vi "GUI_Cascade.vi"() -> ()   [LabVIEW 2013]
uses:
  Shared/GUI_Template/GUI_master/tcp_new_data_event.ctl
  Shared/GUI_Template/GUI_master/tcp new data cluster.ctl
  <vilib>/vision/NI_Vision_Development_Module.lvlib
panel:
  out "Histogram Report":T1 {"Standard  Variation" format="%.2f"; "Mean Value" format="%.2f"; "Interval Width" format="%.2f"; "Starting Value" format="%.2f"; "Maximal Value" format="%.2f"; "Minimal Value" format="%.2f"}
  in  "Number of histogram bins":i32=256
  out "Mean Value":sgl format="%.2f"
  in  "localsavingpath::1":path caption="LocalSavingPath"
  in  "STOP":bool
  out "Lineout":dbl[](graph)
  in  "exposure::1":dbl=40.0 caption="Exposure" min=0.0 max=20000.0
  in  "ADCGain::1":dbl=1.0 caption="ADC Gain" min=0.0 max=2000.0
  in  "AvalancheGain::1":dbl=3000.0 caption="Avalanche Gain" min=0.0 max=10000.0
  in  "Refresh Button":bool
  in  "save::1":bool caption="Save"
  in  "FastADC::1":bool caption="FastADC"
  in  "ROI.Xend::1":dbl=512.0 caption="ROI.Xend" min=1.0 max=512.0
  in  "ROI.Yend::1":dbl=512.0 caption="ROI.Yend" min=1.0 max=512.0
  in  "ROI.Ystart::1":dbl=1.0 caption="ROI.Ystart" min=1.0 max=512.0
  in  "ROI.Xstart::1":dbl=1.0 caption="ROI.Xstart" min=1.0 max=512.0
  in  "ROI.Ybinning::1":dbl=1.0 caption="Y binning" min=1.0 max=512.0
  in  "ROI.Xbinning::1":dbl=1.0 caption="X binning" min=1.0 max=512.0
  in  "trigger::1":T2(ring)=enum."Trigger First (PM only)" caption="Trigger"
  out "image::1":T3(plugin-control) caption="Casca512"
  out "Histogram":T4(graph)
  in  "GUIdevice 1":string="Cascade512"
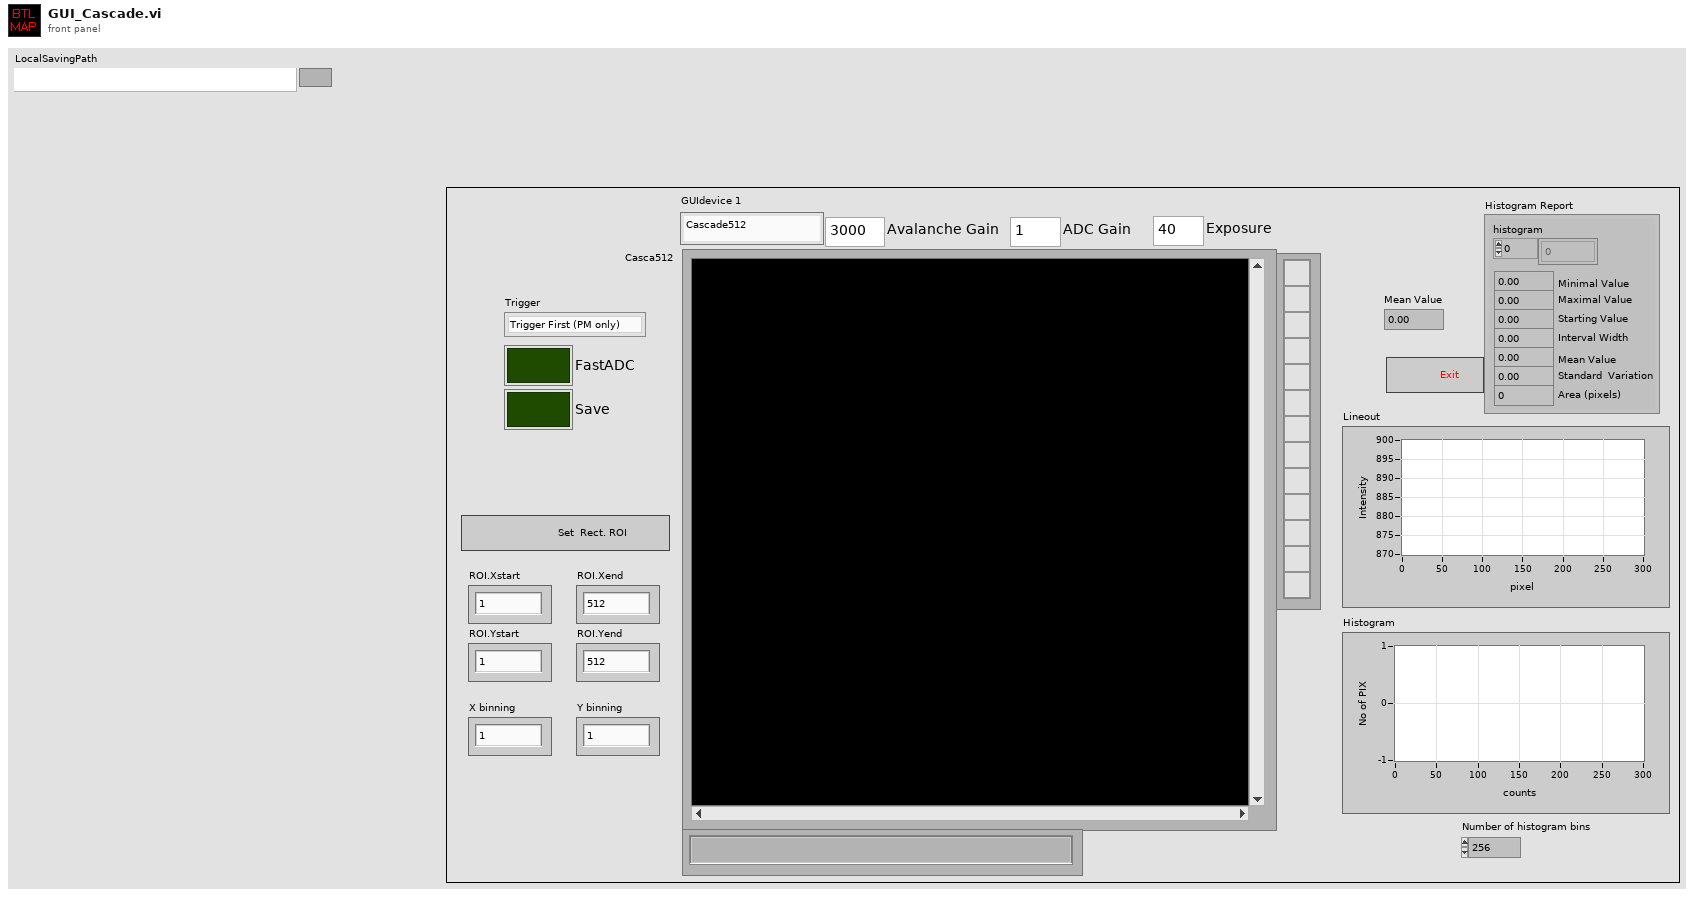
[diagram p1: front panel]
types:
  T1 = cluster{"histogram":u32[], "Minimal Value":sgl, "Maximal Value":sgl, "Starting Value":sgl, "Interval Width":sgl, "Mean Value":sgl, "Standard  Variation":sgl, "Area (pixels)":i32}
  T2 = enum32{"N/A", "Free Run/Timed", "Trigger First (PM only)", "Ext Sync/Strobed", "Bulb (PM only)", "Variable Exp (PM only)", "Flash Mode (PM only)"}
  T3 = typedef "IMAQ Image.ctl" = refnum<image>
  T4 = cluster{"Starting Value":sgl, "Incremental Value":sgl, "Histogram":u32[]}
  T5 = enum32{"invalid app kind", "Development System", "Run Time System", "Student Edition", "Embedded LabVIEW", "Evaluation", "Custom"}
  T6 = typedef "tcp_new_data_event.ctl" = refnum<user-event>
  T7 = typedef "tcp new data cluster.ctl" = cluster{"EventEnum":enum16{"new data", "connection status update"}, "Device name":string}
  T8 = enum32{"Invalid", "Standard", "Closed", "Hidden", "Minimized", "Maximized"}
  T9 = cluster{"Global Rectangle":i32[], "Contours":cluster{"Contour Type":u32, "ROI Type":u32, "Points":i32[]}[]}
  T10 = typedef "IMAQ Line" = cluster{"Start X":i32, "Start Y":i32, "End X":i32, "End Y":i32}
  T11 = typedef "IMAQ Rectangle" = cluster{"Left":i32, "Top":i32, "Right":i32, "Bottom":i32, "Rotation":dbl}
  T12 = cluster{"Core":cluster{"Current VI Reference":refnum<vi>, "Close Panel on Exit?":bool}, "Your Boolean data":bool, "Your string data":string, "SuperGUI":cluster{"STOP queue":refnum<queue>, "SuperGUI ref":refnum<vi>}, "New Image":T3, "tcp data event":T6}
  T13 = typedef "Image Type" = u32
  T14 = cluster{"STOP queue":refnum<queue>, "SuperGUI ref":refnum<vi>}
  T15 = cluster{"Current VI Reference":refnum<vi>, "Close Panel on Exit?":bool}
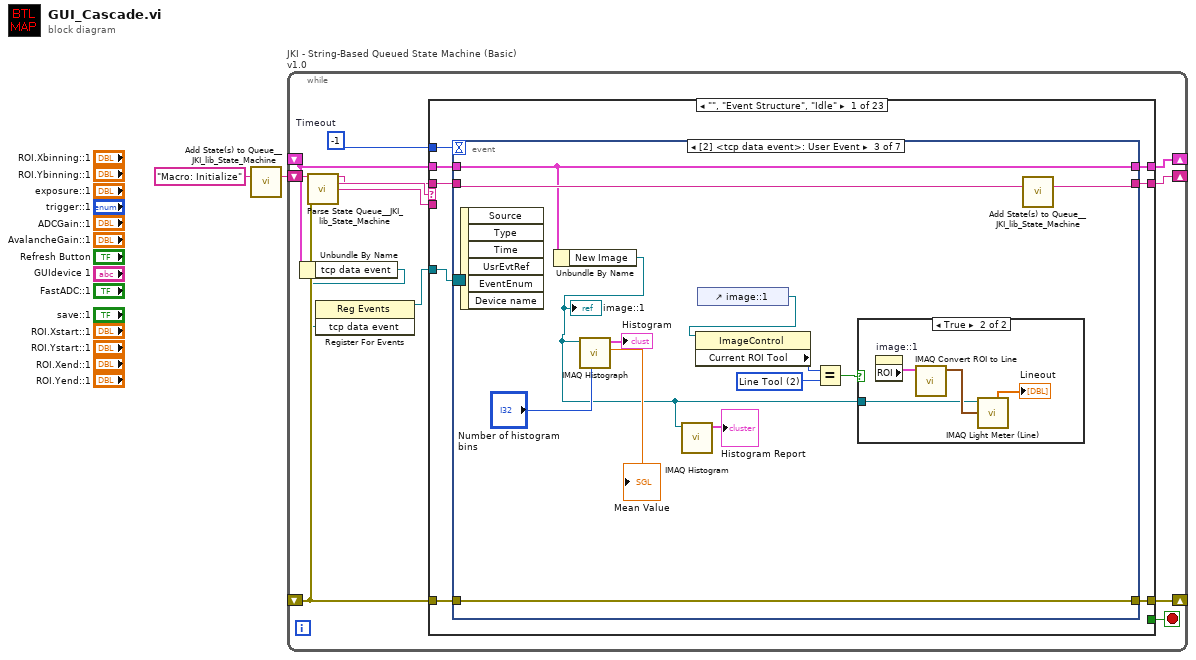
[diagram p0: block diagram]
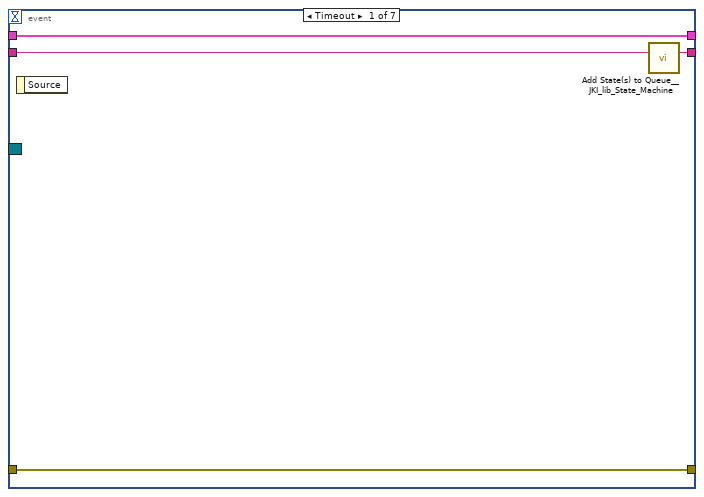
[diagram p2: hidden frame]
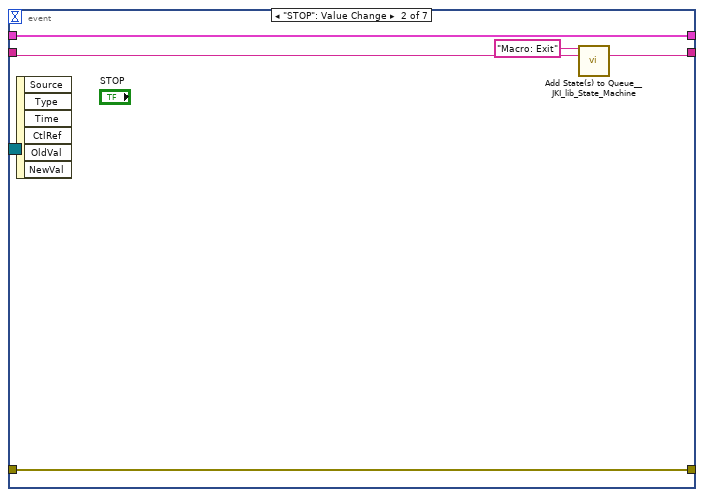
[diagram p3: hidden frame]
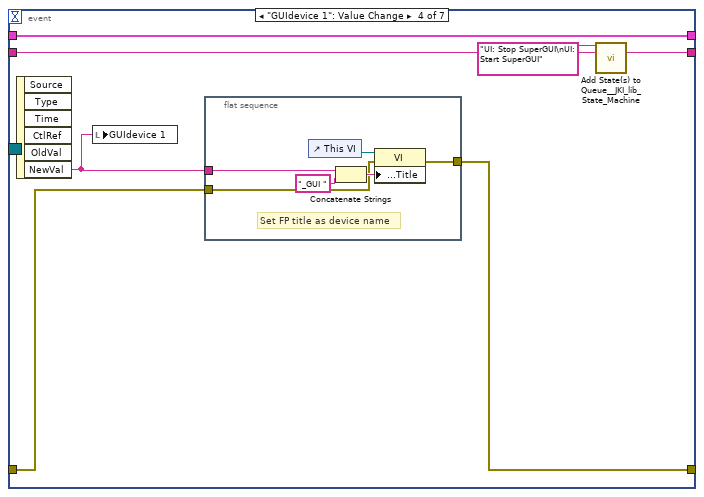
[diagram p5: hidden frame]
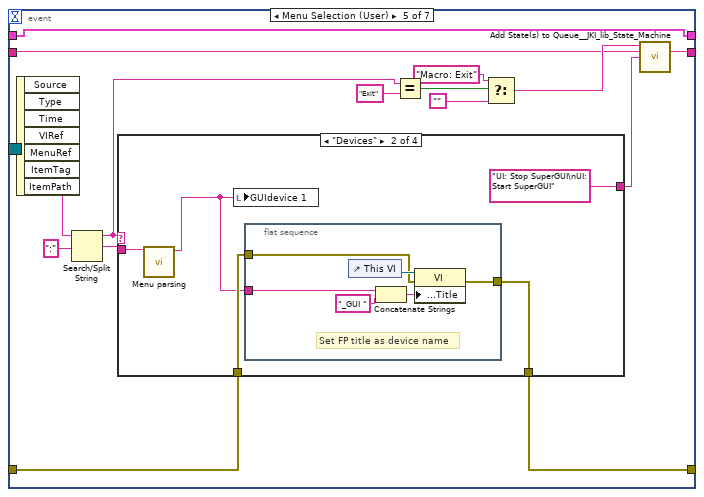
[diagram p6: hidden frame]
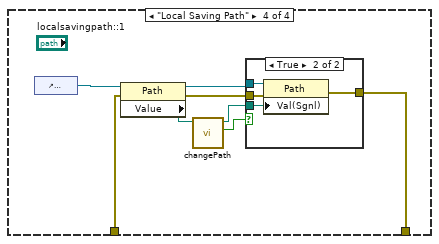
[diagram p9: hidden frame]
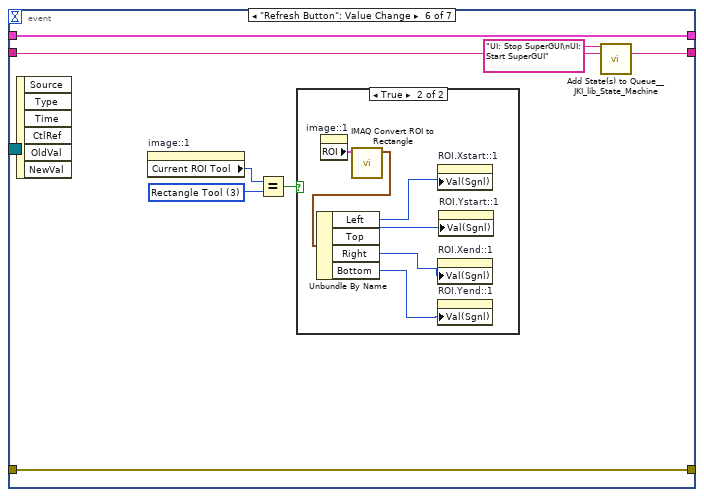
[diagram p11: hidden frame]
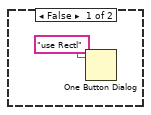
[diagram p12: hidden frame]
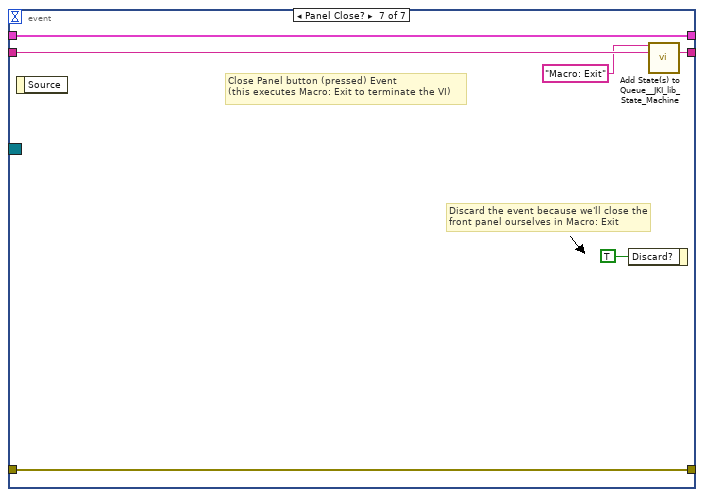
[diagram p13: hidden frame]
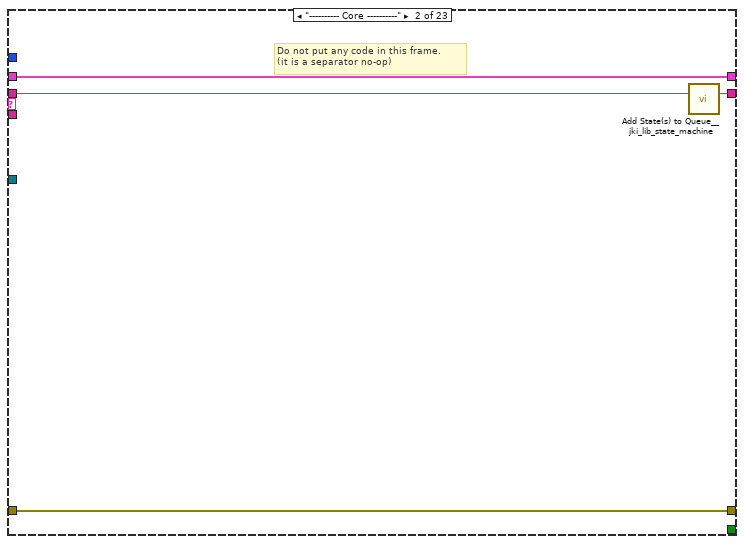
[diagram p14: hidden frame]
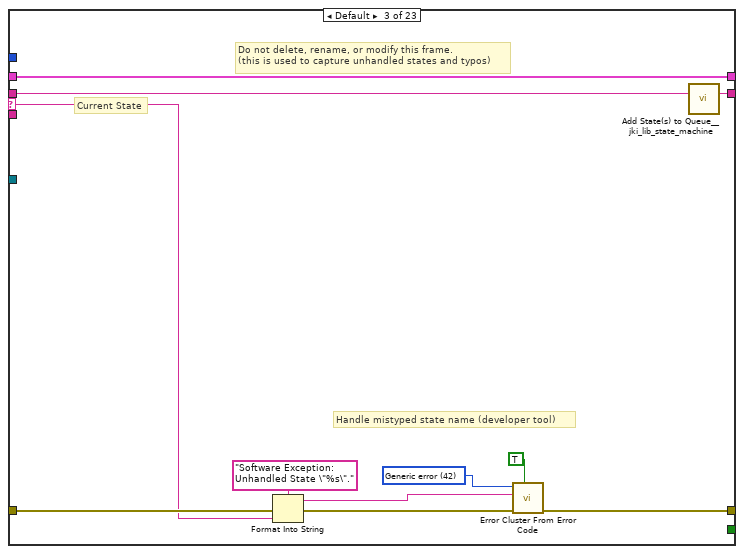
[diagram p15: hidden frame]
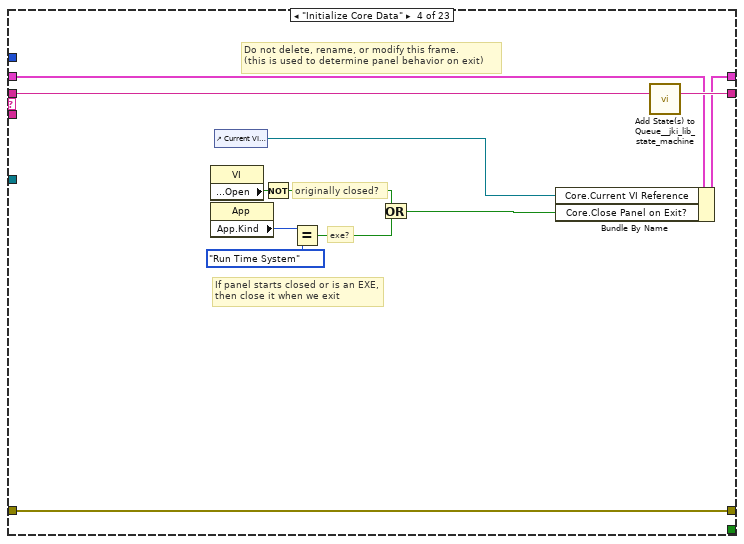
[diagram p16: hidden frame]
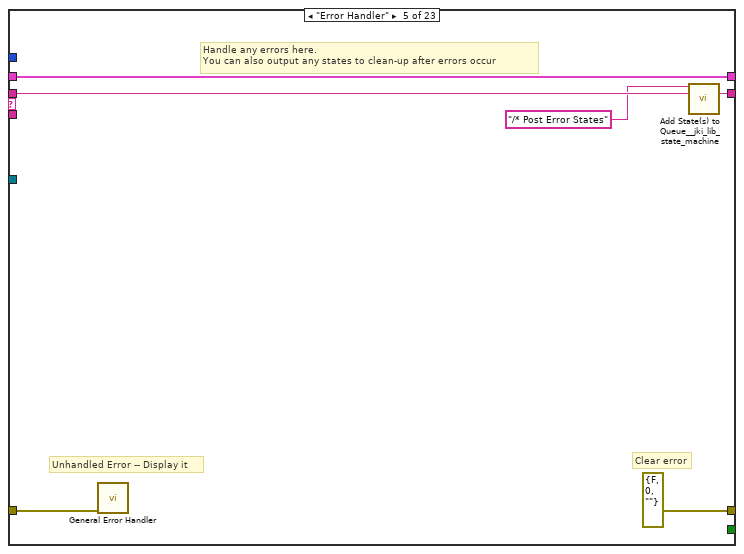
[diagram p17: hidden frame]
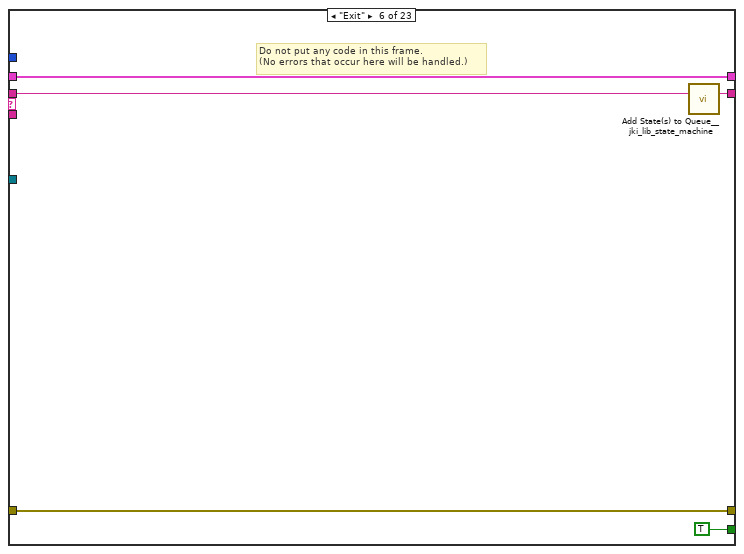
[diagram p18: hidden frame]
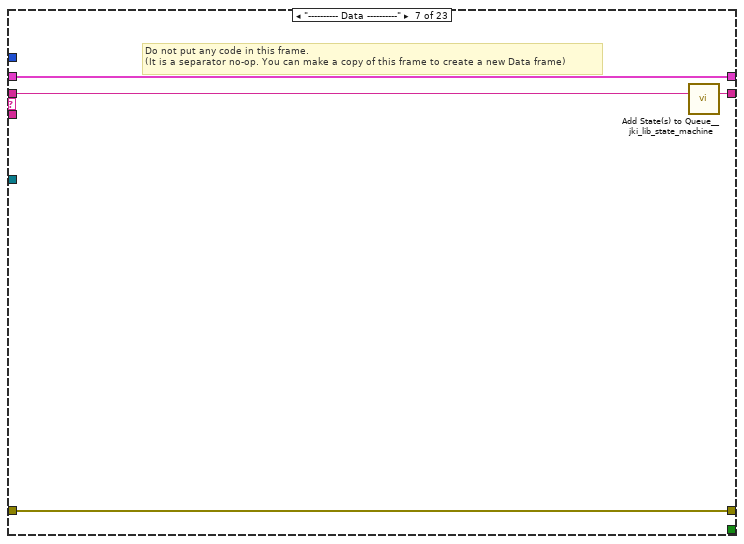
[diagram p19: hidden frame]
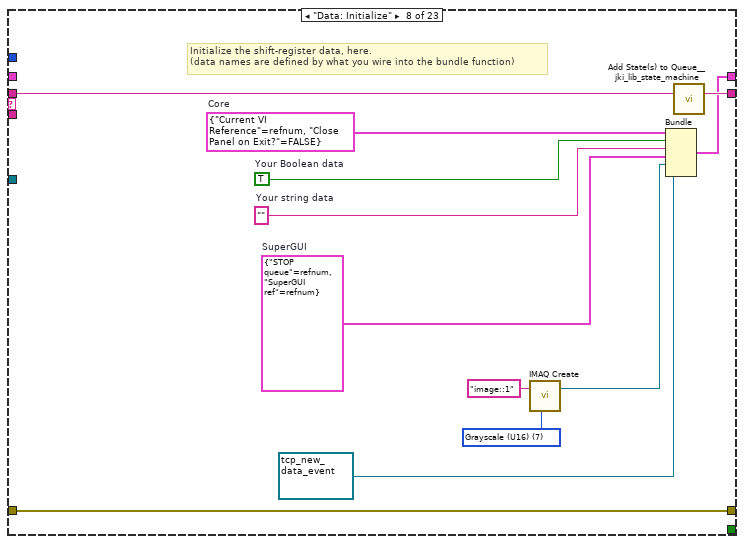
[diagram p20: hidden frame]
diagram:
  n1 = call <vilib>:"Add State(s) to Queue__JKI_lib_State_Machine.vi"("State(s) in (\"\")"="Macro: Initialize") -> ("States Out"=w2:string)  [unwired: 14 in]
  n2 = while "JKI - String-Based Queued State Machine (Basic) v1.0" {
    shift-right: [w8] -> _
    shift-left: _ -> [w5]
    shift-right: [w11] -> _
    shift-left: _ -> [w6]
    shift-right: [w10] -> _
    shift-left: w2 -> [w12]
    stop <- w9 stop-if-true
    w7 = -1  # Timeout
    n3 = Unbundle By Name(w5) -> ("tcp data event"=w4:T6)
    n4 = call <vilib>:"Parse State Queue__JKI_lib_State_Machine.vi"("State Queue"=w12, "Error In (no error)"=w6) -> ("Remaining States"=w14:string, "Current State"=w15:string, "Arguments"=w13:string)  [unwired: 11 in]
    n5 = register-events(w4) -> (reference out=w3:refnum<event-registration>)  [unwired: 2 in, 1 out]
    n6 = case shown="\"\", \"Event Structure\", \"Idle\"" w15 {
      selector: w15 -> [_ _ w129 _ _ _ _ _ _ _ _ _ _ _ _ _ _ _ _ _ _ _ _]
      tunnel: w14 -> [w23 w128 w133 w151 w157 w162 w166 w178 w184 w188 w193 w198 w236 w270 w278 w284 w295 w321 w326 w336 w340 w344 w348]
      tunnel: w13 -> [_ _ _ _ _ _ _ _ _ _ _ _ _ _ _ w279 w289 _ _ _ _ _ _]
      tunnel: w5 -> [w21 w125 w131 w142 w154 w160 w163 _ w179 w185 w191 w196 w234 w261 w273 w282 w291 w318 w323 w333 w337 w341 w345]
      tunnel: [w20 w126 w135 w148 errorcluster {"status"=FALSE, "code"=0, "source"=""} ("error out") w159 w164 w175 w180 w186 w189 w194 w231 w255 w271 w280 w292 w319 w324 w334 w338 w342 w346] -> w11
      tunnel: w6 -> [w19 w126 w134 w148 w153 w159 w164 w175 w181 w186 w190 w195 w232 w256 w272 w281 w293 w319 w324 w334 w338 w342 w346]
      tunnel: [w22 w127 w132 w150 w156 w161 w165 w177 w183 w187 w192 w197 w235 w269 w277 w283 w294 w320 w325 w335 w339 w343 w347] -> w10
      tunnel: [_ _ _ _ _ TRUE _ _ _ _ _ _ _ _ _ _ _ _ _ _ _ _ _] -> w9
      tunnel: [w18 w125 w131 w149 w154 w160 w163 w176 w179 w185 w191 w196 w234 w260 w273 w282 w291 w318 w323 w333 w337 w341 w345] -> w8
      tunnel: w7 -> [w17 _ _ _ _ _ _ _ _ _ _ _ _ _ _ _ _ _ _ _ _ _ _]
      tunnel: w3 -> [w16 _ _ _ _ _ _ _ _ _ _ _ _ _ _ _ _ _ _ _ _ _ _]
      frame "", "Event Structure", "Idle" {
        n7 = event shown="[2] <tcp data event>: User Event" {
          selector: w16 -> [_ _ _ _ _ _ _]
          dyn-events: _ -> [_ _ _ _ _ _ _]
          timeout: w17 -> [_ _ _ _ _ _ _]
          tunnel: w23 -> [w27 w30 w44 w53 w71 w109 w124]
          tunnel: [w26 w29 w43 w52 w70 w108 w123] -> w22
          tunnel: w21 -> [w24 w32 w38 w56 w77 w111 w121]
          tunnel: [w25 w31 w45 w54 w64 w110 w122] -> w20
          tunnel: w19 -> [w25 w31 w45 w55 w65 w110 w122]
          tunnel: [w24 w32 w38 w56 w77 w111 w121] -> w18
          event Timeout {
            n8 = event-data() -> ()  [unwired: 1 in, 1 out]
            n9 = call <vilib>:"Add State(s) to Queue__JKI_lib_State_Machine.vi"("State(s) in (\"\")"=w27) -> ("States Out"=w26:string)  [unwired: 14 in]
          }
          event "STOP": Value Change {
            n10 = event-data() -> ()  [unwired: 1 in, 6 out]
            n11 = call <vilib>:"Add State(s) to Queue__JKI_lib_State_Machine.vi"("State(s) in Front (\"\")"="Macro: Exit", "State(s) in (\"\")"=w30) -> ("States Out"=w29:string)  [unwired: 13 in]
          }
          event User Event {
            w41 = u32 2 items=["Zoom Tool"=8, "Selection Tool"=0, "Pan Tool"=9, "Point Tool"=1, "Line Tool"=2, "Rectangle Tool"=3, "Rotated Rectangle Tool"=12, "Polyline Tool"=10, "Polygon Tool"=5, "Freehand Tool"=11, "Closed Freehand Tool"=6, "Ellipse Tool"=4, "Annulus Tool"=7] ("Current ROI Tool")
            n12 = event-data() -> ()  [unwired: 1 in, 6 out]
            n13 = Unbundle By Name(w38) -> ("New Image"=w34:T3)
            "image::1" <- w34
            n14 = call "IMAQ Histograph"("Number of Classes"="Number of histogram bins", "Image"=w34) -> ("Mean Value"=→"Mean Value":sgl, "Histogram Graph"=→"Histogram":T4)  [unwired: 6 in, 2 out]
            n15 = call "IMAQ Histogram"("Image"=w34) -> ("Histogram Report"=→"Histogram Report":T1)  [unwired: 9 in, 1 out]
            n16 = control-ref of="image::1"() -> (w37:refnum<vi>)
            n17 = property on="Property Node" class="ImageControl"(reference=w37) -> ("Current ROI Tool"=w40:u32)  [unwired: 1 in, 2 out]
            n18 = Equal?(x=w40, y=w41) -> (x = y?=w42:bool)
            n19 = case shown="True" w42 {
              tunnel: w34 -> [_ w47]
              frame False {
              }
              frame True {
                n20 = property on="image::1" class="ImageControl"() -> ("ROI"=w49:T9)  [unwired: 2 in, 2 out]
                n21 = call "IMAQ Convert ROI to Line"("ROI Descriptor"=w49) -> ("Line"=w48:T10)  [unwired: 8 in, 1 out]
                n22 = call "IMAQ Light Meter (Line)"("Line"=w48, "Image"=w47) -> ("Line Profile"=→"Lineout":dbl[])  [unwired: 5 in, 4 out]
              }
            }
            n23 = call <vilib>:"Add State(s) to Queue__JKI_lib_State_Machine.vi"("State(s) in (\"\")"=w44) -> ("States Out"=w43:string)  [unwired: 14 in]
          }
          event "GUIdevice 1": Value Change {
            n24 = event-data() -> ("NewVal"=w50:string)  [unwired: 1 in, 5 out]
            n25 = local write "GUIdevice 1"(w50) -> ()
            n26 = flat-sequence {
              tunnel: [w59] -> w54
              tunnel: w55 -> [w58]
              tunnel: w50 -> [w57]
              frame #0 {
                # "Set FP title as device name"
                n27 = control-ref of="This VI"() -> (w62:refnum<vi>)
                n28 = Concatenate Strings(w57, "_GUI ") -> (w61:string)
                n29 = property class="VI"(reference=w62, error in=w58, "Front Panel.Title"=w61) -> (error out=w59:errorcluster)  [unwired: 1 out]
              }
            }
            n30 = call <vilib>:"Add State(s) to Queue__JKI_lib_State_Machine.vi"("State(s) in Front (\"\")"="UI: Stop SuperGUI\nUI: Start SuperGUI", "State(s) in (\"\")"=w53) -> ("States Out"=w52:string)  [unwired: 13 in]
          }
          event Menu Selection (User) {
            n31 = event-data() -> ("ItemPath"=w67:string)  [unwired: 1 in, 6 out]
            n32 = Search/Split String(string=w67, search string/char (-)=":") -> (substring before match=w63:string, match + rest of string=w66:string)  [unwired: 1 in, 1 out]
            n33 = case shown="\"Devices\"" w63 {
              tunnel: w66 -> [_ w83 _ _]
              tunnel: w65 -> [w78 w82 w90 w93]
              tunnel: [w78 w81 w90 w92] -> w64
              tunnel: [_ "UI: Stop SuperGUI\nUI: Start SuperGUI" _ _] -> w69
              frame "", Default {
              }
              frame "Devices" {
                n34 = call "Menu parsing.vi"("ItemPath"=w83) -> ("ItemPath"=w79:string)  [unwired: 9 in, 1 out]
                n35 = local write "GUIdevice 1"(w79) -> ()
                n36 = flat-sequence {
                  tunnel: [w86] -> w81
                  tunnel: w82 -> [w85]
                  tunnel: w79 -> [w84]
                  frame #0 {
                    # "Set FP title as device name"
                    n37 = control-ref of="This VI"() -> (w89:refnum<vi>)
                    n38 = Concatenate Strings(w84, "_GUI ") -> (w88:string)
                    n39 = property class="VI"(reference=w89, error in=w85, "Front Panel.Title"=w88) -> (error out=w86:errorcluster)  [unwired: 1 out]
                  }
                }
              }
              frame "Exit" {
              }
              frame "Local Saving Path" {
                n40 = control-ref of="localsavingpath::1"() -> (w94:refnum<vi>)
                n41 = property class="Path"(reference=w94, error in=w93) -> (reference out=w96:refnum<vi>, error out=w91:errorcluster, "Value"=w95:path)
                n42 = call "changePath.vi"("Local Saving in (h)"=w95) -> ("change (h)"=w97:bool, "Local Saving out (h)"=w98:path)  [unwired: 9 in]
                n43 = case shown="True" w97 {
                  tunnel: w96 -> [_ w103]
                  tunnel: w98 -> [_ w102]
                  tunnel: [w99 w101] -> w92
                  tunnel: w91 -> [w99 w100]
                  frame False {
                  }
                  frame True {
                    n44 = property class="Path"(reference=w103, error in=w100, "Val(Sgnl)"=w102) -> (error out=w101:errorcluster)  [unwired: 1 out]
                  }
                }
              }
            }
            n45 = Equal?(x=w63, y="Exit") -> (x = y?=w75:bool)
            n46 = Select(t="Macro: Exit", s=w75, f="") -> (s? t:f=w72:string)
            n47 = call <vilib>:"Add State(s) to Queue__JKI_lib_State_Machine.vi"("State(s) in Front (\"\")"=w72, "State(s) in (\"\")"=w71, "State(s) at Back (\"\")"=w69) -> ("States Out"=w70:string)  [unwired: 12 in]
          }
          event "Refresh Button": Value Change {
            w105 = u32 3 items=["Zoom Tool"=8, "Selection Tool"=0, "Pan Tool"=9, "Point Tool"=1, "Line Tool"=2, "Rectangle Tool"=3, "Rotated Rectangle Tool"=12, "Polyline Tool"=10, "Polygon Tool"=5, "Freehand Tool"=11, "Closed Freehand Tool"=6, "Ellipse Tool"=4, "Annulus Tool"=7] ("Current ROI Tool")
            n48 = event-data() -> ()  [unwired: 1 in, 6 out]
            n49 = property on="image::1" class="ImageControl"() -> ("Current ROI Tool"=w106:u32)  [unwired: 2 in, 2 out]
            n50 = Equal?(x=w106, y=w105) -> (x = y?=w104:bool)
            n51 = case shown="True" w104 {
              frame False {
                n52 = One Button Dialog(message="use Rectl") -> ()  [unwired: 1 in, 1 out]
              }
              frame True {
                n53 = property on="image::1" class="ImageControl"() -> ("ROI"=w118:T9)  [unwired: 2 in, 2 out]
                n54 = call "IMAQ Convert ROI to Rectangle"("ROI Descriptor"=w118) -> ("Rectangle"=w117:T11)  [unwired: 8 in, 1 out]
                n55 = Unbundle By Name(w117) -> ("Left"=w116:i32, "Top"=w115:i32, "Right"=w114:i32, "Bottom"=w113:i32)
                n56 = property on="ROI.Xstart::1" class="DigNum (strict)"("Val(Sgnl)"=w116) -> ()  [unwired: 2 in, 2 out]
                n57 = property on="ROI.Xend::1" class="DigNum (strict)"("Val(Sgnl)"=w114) -> ()  [unwired: 2 in, 2 out]
                n58 = property on="ROI.Yend::1" class="DigNum (strict)"("Val(Sgnl)"=w113) -> ()  [unwired: 2 in, 2 out]
                n59 = property on="ROI.Ystart::1" class="DigNum (strict)"("Val(Sgnl)"=w115) -> ()  [unwired: 2 in, 2 out]
              }
            }
            n60 = call <vilib>:"Add State(s) to Queue__JKI_lib_State_Machine.vi"("State(s) in Front (\"\")"="UI: Stop SuperGUI\nUI: Start SuperGUI", "State(s) in (\"\")"=w109) -> ("States Out"=w108:string)  [unwired: 13 in]
          }
          event Panel Close? {
            # "Discard the event because we'll close the front panel ourselves in Macro: Exit"
            # "Close Panel button (pressed) Event\n(this executes Macro: Exit to terminate the VI)"
            n61 = event-data() -> ()  [unwired: 1 in, 1 out]
            n62 = event-data("Discard?"=TRUE) -> ()  [unwired: 1 in, 1 out]
            n63 = call <vilib>:"Add State(s) to Queue__JKI_lib_State_Machine.vi"("State(s) in Front (\"\")"="Macro: Exit", "State(s) in (\"\")"=w124) -> ("States Out"=w123:string)  [unwired: 13 in]
          }
        }
      }
      frame "---------- Core ----------" {
        # "Do not put any code in this frame.\n(it is a separator no-op)"
        n64 = call <vilib>:"Add State(s) to Queue__jki_lib_state_machine.vi"("State(s) in (\"\")"=w128) -> ("States Out"=w127:string)  [unwired: 14 in]
      }
      frame Default {
        w138 = 42 items=["No error", "Argument error", "Memory is full", "Out of zone", "End of file", "File already open", "Generic file I/O error", "File not found", "File permission error", "Disk is full", "Duplicate path", "Too many files open", "System feature not enabled", "Resource file not found", "Cannot add resource", "Resource not found", "Image not found", "Image memory error", "Pen does not exist", "Config type invalid", "Config token not found", "Config parse error", "Config memory error", "Bad external code format", "Bad external code offset", "External code not present", "Null window", "Destroy window error", "Null menu", "Print aborted", "Bad print record", "Print driver error", "Windows error during printing", "Memory error during printing", "Print dialog error", "Generic print error", "Invalid device refnum", "Device not found", "Device parameter error", "Device unit error", "Cannot open device", "Device call aborted", "Generic error", "Cancelled by user", "Object ID too low", "Object ID too high", "Object not in heap", "Unknown heap", "Unknown object (invalid DefProc)", "Unknown object (DefProc not in table)", "Message out of range", "Invalid (null) method", "Unknown message", "Manager call not supported", "Bad address", "Network operation in progress", "Network operation timed out", "Connection is busy", "Network attribute not supported", "Network error", "Address in use", "System out of memory", "Connection aborted", "Connection refused", "Not connected", "Already connected", "Connection closed", "Initialization error (interapplication manager)", "Bad occurrence", "Wait on unbound occurrence handler", "Occurrence queue overflow", "Datalog type conflict", "Unused", "Unrecognized type (interapplication manager)", "Memory corrupt", "Failed to make temporary DLL", "Old CIN version", "Drag socket not found", "Failed to load drop-object", "Failed to register OLE object", "Failed to release OLE object", "Format specifier type mismatch", "Unknown format specifier", "Too few format specifiers", "Too many format specifiers", "Scan failed", "Newer CIN version", "Error converting to variant", "Runtime menu error", "Password tampered", "Variant attribute not found", "Incompatible variant data type", "Event data is not available", "Event Store is not present", "Occurrence is not found", "Event Queue is not created", "Event info is not available", "Refnum passed is NULL", "Error retrieving Class GUID", "Error retrieving CoClass GUID", "Error retrieving TypeLib GUID.", "Bad built application magic bytes.", "Specific driver is different from the specific driver associated with the Logical Name.", "There is no session opened to the class driver.", "Max Error", "MAX - Error with config objects", "MAX - Error loading configuration", "MAX - Group not supported"]
        # "Current State"
        # "Do not delete, rename, or modify this frame.\n(this is used to capture unhandled states and typos)"
        # "Handle mistyped state name (developer tool)"
        n65 = Format Into String(format string="Software Exception: Unhandled State \"%s\"." ("message"), error in=w134, w129) -> (resulting string=w137:string, error out=w136:errorcluster)  [unwired: 1 in]
        n66 = call <vilib>:"Error Cluster From Error Code.vi"("show call chain? (False)"=TRUE, "error in (no error)"=w136, "error message (\"\")"=w137, "error code (0)"=w138) -> ("error out"=w135:errorcluster)  [unwired: 5 in]
        n67 = call <vilib>:"Add State(s) to Queue__jki_lib_state_machine.vi"("State(s) in (\"\")"=w133) -> ("States Out"=w132:string)  [unwired: 14 in]
      }
      frame "Initialize Core Data" {
        # "Do not delete, rename, or modify this frame.\n(this is used to determine panel behavior on exit)"
        # "originally closed?"
        # "exe?"
        # "If panel starts closed or is an EXE, then close it when we exit"
        n68 = property class="VI"() -> ("Front Panel.Open"=w147:bool)  [unwired: 2 in, 2 out]
        n69 = property class="App"() -> ("App.Kind"=w146:T5)  [unwired: 2 in, 2 out]
        n70 = control-ref of="Current VI Reference"() -> (w140:refnum<vi>)
        n71 = Not(x=w147) -> (.not. x?=w144:bool)
        n72 = Equal?(x=w146, y=T5."Run Time System" ("Application:Kind")) -> (x = y?=w143:bool)
        n73 = Or(x=w144, y=w143) -> (x .or. y?=w141:bool)
        n74 = Bundle By Name(cluster=w142, "Core.Current VI Reference"=w140, "Core.Close Panel on Exit?"=w141) -> (w149:T12)
        n75 = call <vilib>:"Add State(s) to Queue__jki_lib_state_machine.vi"("State(s) in (\"\")"=w151) -> ("States Out"=w150:string)  [unwired: 14 in]
      }
      frame "Error Handler" {
        # "Unhandled Error -- Display it"
        # "Handle any errors here.\nYou can also output any states to clean-up after errors occur"
        # "Clear error"
        n76 = call <vilib>:"General Error Handler.vi"("error in (no error)"=w153) -> ()  [unwired: 10 in, 5 out]
        n77 = call <vilib>:"Add State(s) to Queue__jki_lib_state_machine.vi"("State(s) in Front (\"\")"="/* Post Error States", "State(s) in (\"\")"=w157) -> ("States Out"=w156:string)  [unwired: 13 in]
      }
      frame "Exit" {
        # "Do not put any code in this frame.\n(No errors that occur here will be handled.)"
        n78 = call <vilib>:"Add State(s) to Queue__jki_lib_state_machine.vi"("State(s) in (\"\")"=w162) -> ("States Out"=w161:string)  [unwired: 14 in]
      }
      frame "---------- Data ----------" {
        # "Do not put any code in this frame.\n(It is a separator no-op. You can make a copy of this frame to create a new Data frame)"
        n79 = call <vilib>:"Add State(s) to Queue__jki_lib_state_machine.vi"("State(s) in (\"\")"=w166) -> ("States Out"=w165:string)  [unwired: 14 in]
      }
      frame "Data: Initialize" {
        w170 = T13 7 items=["Grayscale (U8)", "Grayscale (I16)", "Grayscale (SGL)", "Complex (CSG)", "RGB (U32)", "HSL (U32)", "RGB (U64)", "Grayscale (U16)"] ("Image Type")
        w171 = T14 {"STOP queue"=refnum, "SuperGUI ref"=refnum}  # SuperGUI
        w172 = T15 {"Current VI Reference"=refnum, "Close Panel on Exit?"=FALSE}  # Core
        w174 = TRUE  # Your Boolean data
        w173 = ""  # Your string data
        # "Initialize the shift-register data, here.\n(data names are defined by what you wire into the bundle function)"
        n80 = call "IMAQ Create"("Image Name"="image::1", "Image Type"=w170) -> ("New Image"=w168:T3)  [unwired: 3 in, 1 out]
        n81 = Bundle("Core"=w172, "Your Boolean data"=w174, "Your string data"=w173, "SuperGUI"=w171, "New Image"=w168, "tcp data event"=T6 refnum) -> (w176:T12)  [unwired: 1 in]
        n82 = call <vilib>:"Add State(s) to Queue__jki_lib_state_machine.vi"("State(s) in (\"\")"=w178) -> ("States Out"=w177:string)  [unwired: 14 in]
      }
      frame "Data: Cleanup" {
        # "Cleanup any data and references, here.\n(this is called automatically, by the Macro: Exit)"
        n83 = Unbundle By Name(w179) -> ("Core.Current VI Reference"=w182:refnum<vi>)
        n84 = Close Reference(reference=w182, error in (no error)=w181) -> (error out=w180:errorcluster)
        n85 = call <vilib>:"Add State(s) to Queue__jki_lib_state_machine.vi"("State(s) in (\"\")"=w184) -> ("States Out"=w183:string)  [unwired: 14 in]
      }
      frame "---------- UI ----------" {
        # "Do not put any code in this frame.\n(It is a separator no-op. You can make a copy of this frame to create a new UI frame)"
        n86 = call <vilib>:"Add State(s) to Queue__jki_lib_state_machine.vi"("State(s) in (\"\")"=w188) -> ("States Out"=w187:string)  [unwired: 14 in]
      }
      frame "UI: Initialize" {
        # "Initialize the User Interface, here.\n(this is called automatically, by the Macro: Init)"
        n87 = call <userlib>:"Fit VI window to Largest Dec__ogtk.vi"("error in (no error)"=w190) -> ("error out"=w189:errorcluster)  [unwired: 5 in, 1 out]
        n88 = call <vilib>:"Add State(s) to Queue__jki_lib_state_machine.vi"("State(s) in (\"\")"=w193) -> ("States Out"=w192:string)  [unwired: 14 in]
      }
      frame "UI: Update Device List" {
        n89 = disable-structure shown="Disabled" {
          disable-tunnel: w195 -> [w203 w230]
          disable-tunnel: [w201 w230] -> w194
          frame Disabled {
            n90 = call "getDevices.vi"("Device Class"="FROG") -> ("All Devices"=w199:string[])
            n91 = Empty Array?(array=w199) -> (empty?=w200:bool)
            n92 = case shown="False" w200 {
              tunnel: w203 -> [w206 w229]
              tunnel: [w205 w229] -> w201
              tunnel: w199 -> [w204 _]
              frame False {
                n93 = Current VI's Menubar() -> (w209:refnum<k9>)
                n94 = Get Menu Item Info(7:"Devices" ("item tag"), 8:w206, 11:w209) -> (0:w215:errorcluster, 3:w211:refnum<k9>)  [unwired: 5 out]
                n95 = Set Menu Item Info(7:"Devices" ("item tag"), 8:w215, 9:TRUE ("enabled"), 11:w211) -> (0:w214:errorcluster, 3:w213:refnum<k9>)  [unwired: 3 in]
                n96 = First Call?() -> (First Call?: T/F=w207:bool)
                n97 = case shown="True" w207 {
                  tunnel: w213 -> [_ w221]
                  tunnel: w204 -> [_ w220]
                  tunnel: w214 -> [w216 w218]
                  tunnel: [w216 w217] -> w205
                  frame False {
                  }
                  frame True {
                    n98 = for {
                      tunnel: [w228] -> w222
                      tunnel: w220 -> [w226] mode=indexing
                      tunnel: w221 -> [w225]
                      tunnel: [w224] -> w219
                      tunnel: w218 -> [w223]
                      n99 = Insert Menu Items(5:"Devices" ("menu tag"), 6:w223, 7:w226, 8:w226, 9:w225) -> (0:w224:errorcluster, 3:w228:refnum<k9>)  [unwired: 1 in, 1 out]
                    }
                    n100 = Enable Menu Tracking(2:w219, 4:w222) -> (0:w217:errorcluster)  [unwired: 1 in, 1 out]
                  }
                }
              }
              frame True {
              }
            }
          }
          frame Enabled {
          }
        }
        n101 = call <vilib>:"Add State(s) to Queue__jki_lib_state_machine.vi"("State(s) in (\"\")"=w198) -> ("States Out"=w197:string)  [unwired: 14 in]
      }
      frame "UI: Get Device Name" {
        n102 = First Call?() -> (First Call?: T/F=w233:bool)
        n103 = case shown="True" w233 {
          tunnel: w232 -> [w237 w239]
          tunnel: [w237 w238] -> w231
          frame False {
          }
          frame True {
            n104 = disable-structure "Get Device name from control for vi mode\nand command line arg for exe" shown="RUN_TIME_ENGINE==True" {
              disable-tunnel: w239 -> [_ w241]
              disable-tunnel: [_ w240] -> w238
              frame condition #0 (active) {
              }
              frame condition #1 {
                n105 = control-ref of="This Application"() -> (w249:refnum<vi>)
                n106 = property class="App"(reference=w249) -> ("App.Args"=w248:string[])  [unwired: 1 in, 2 out]
                n107 = Index Array(array=w248, index #1=1 ("index")) -> (element #1=w242:string)  [unwired: 2 in, 2 out]
                n108 = Empty String/Path?(string/path=w242) -> (empty?=w246:bool)
                n109 = control-ref of="This VI"() -> (w245:refnum<vi>)
                n110 = case shown="False" w246 {
                  tunnel: w242 -> [w250 _]
                  frame False {
                    n111 = local write "GUIdevice 1"(w250) -> ()
                  }
                  frame True {
                  }
                }
                n112 = Concatenate Strings(w242, "_GUI ") -> (w244:string)
                n113 = property class="VI"(reference=w245, error in=w241, "Front Panel.Title"=w244) -> (error out=w240:errorcluster)  [unwired: 1 out]
              }
            }
          }
        }
        n114 = call <vilib>:"Add State(s) to Queue__jki_lib_state_machine.vi"("State(s) in (\"\")"=w236) -> ("States Out"=w235:string)  [unwired: 14 in]
      }
      frame "UI: Start SuperGUI" {
        # "create stop queue for supergui and its clones"
        # "x100 abort will be dependent on caller VI\nx80 abort will be independent of caller vi, this will abort vi when labview is closed."
        # "Start SuperGUI asynchronous way"
        n115 = vi-ref "GUI_Master_subvi_reentrant_queues.vi"() -> (w254:refnum<vi>)
        n116 = property class="VI"(reference=w254) -> ("Path"=w253:path)  [unwired: 1 in, 2 out]
        n117 = Create User Event(user event datatype=T7 {"EventEnum"=enum."new data", "Device name"="Device name"} ("New Event"), error in=w256) -> (user event=w251:refnum<user-event>, error out=w262:errorcluster)
        n118 = control-ref of="This Application"() -> (w259:refnum<vi>)
        n119 = control-ref of="This VI"() -> (w258:refnum<vi>)
        n120 = Open VI Reference(type specifier VI Refnum (for type only)=refnum<vi> refnum, vi path=w253, options=256) -> (vi reference=w268:refnum<vi>, error out=w267:errorcluster)  [unwired: 3 in]
        n121 = register-events(w251) -> ()  [unwired: 2 in, 2 out]
        n122 = call "supergui create stop queue.vi"() -> ("STOP Queue out"=w264:refnum<queue>)  [unwired: 11 in]
        n123 = Current VI's Menubar() -> (w257:refnum<k9>)
        n124 = call-by-ref "Start Asynchronous Call"(reference=w268, error in=w267, "STOP Queue in"=w264, "This Application"=w259, 8:"error in (no error)"=w262, "tcp data event"=w251, "Caller menu reference"=w257, "Caller VI ref"=w258) -> (reference out=w252:refnum<vi>, error out=w255:errorcluster)  [unwired: 5 in, 1 out]
        n125 = Bundle By Name(cluster=w261, "tcp data event"=w251, "SuperGUI.SuperGUI ref"=w252, "SuperGUI.STOP queue"=w264) -> (w260:T12)
        n126 = call <vilib>:"Add State(s) to Queue__jki_lib_state_machine.vi"("State(s) in (\"\")"=w270) -> ("States Out"=w269:string)  [unwired: 14 in]
      }
      frame "UI: Stop SuperGUI" {
        # "Stop Supergui Clone and wait until it exit properly"
        n127 = Unbundle By Name(w273) -> ("SuperGUI.SuperGUI ref"=w275:refnum<vi>, "SuperGUI.STOP queue"=w274:refnum<queue>)
        n128 = Release Queue(queue=w274, error in (no error)=w272) -> (error out=w276:errorcluster)  [unwired: 1 in, 2 out]
        n129 = call-by-ref "Wait On Asynchronous Call"(reference=w275, error in=w276) -> ("error out"=w271:errorcluster)  [unwired: 11 in, 2 out]
        n130 = call <vilib>:"Add State(s) to Queue__jki_lib_state_machine.vi"("State(s) in (\"\")"=w278) -> ("States Out"=w277:string)  [unwired: 14 in]
      }
      frame "UI: Cursor Set" {
        # "Argument"
        # "Set and Unset Cursor Busy.\n(Usage: \"UI: Cursor Set >> Busy|Idle\")"
        n131 = case shown="\"Idle\", Default" w279 {
          tunnel: w281 -> [w286 w288]
          tunnel: [w285 w287] -> w280
          frame "Idle", Default {
            n132 = call <vilib>:"Unset Busy.vi"("error in (no error)"=w286) -> ("error out"=w285:errorcluster)  [unwired: 10 in]
          }
          frame "Busy" {
            n133 = call <vilib>:"Set Busy.vi"("error in (no error)"=w288) -> ("error out"=w287:errorcluster)  [unwired: 9 in, 1 out]
          }
        }
        n134 = call <vilib>:"Add State(s) to Queue__jki_lib_state_machine.vi"("State(s) in (\"\")"=w284) -> ("States Out"=w283:string)  [unwired: 14 in]
      }
      frame "UI: Front Panel State" {
        # "Argument"
        # "Set Front Panel Open or Closed\n(Usage: \"UI: Front Panel State >> Open|Close\")"
        n135 = Unbundle By Name(w291) -> ("Core.Current VI Reference"=w290:refnum<vi>)
        n136 = case shown="\"Open\", Default" w289 {
          tunnel: w293 -> [w299 w312]
          tunnel: [w301 w313] -> w292
          tunnel: w290 -> [w300 w310]
          frame "Open", Default {
            n137 = property class="VI"(reference=w300, error in=w299) -> (reference out=w297:refnum<vi>, error out=w298:errorcluster, "Front Panel.Open"=w296:bool)
            n138 = case shown="False" w296 {
              tunnel: [w304 w307] -> w301
              tunnel: w298 -> [w303 w307]
              tunnel: w297 -> [w302 _]
              frame False {
                n139 = invoke class="VI" method="FP.Open"(reference=w302, error in=w303, "Activate"=TRUE, "State"=T8."Standard") -> (error out=w304:errorcluster)  [unwired: 1 in, 4 out]
              }
              frame True {
              }
            }
          }
          frame "Close" {
            n140 = property class="VI"(reference=w310, error in=w312) -> (reference out=w309:refnum<vi>, error out=w311:errorcluster, "Front Panel.Open"=w308:bool)
            n141 = case shown="True" w308 {
              tunnel: [w314 w317] -> w313
              tunnel: w311 -> [w314 w316]
              tunnel: w309 -> [_ w315]
              frame False {
              }
              frame True {
                n142 = invoke class="VI" method="FP.Close"(reference=w315, error in=w316) -> (error out=w317:errorcluster)  [unwired: 1 in, 2 out]
              }
            }
          }
        }
        n143 = call <vilib>:"Add State(s) to Queue__jki_lib_state_machine.vi"("State(s) in (\"\")"=w295) -> ("States Out"=w294:string)  [unwired: 14 in]
      }
      frame "---------- Macro ----------" {
        # "Do not put any code in this frame.\n(It is a separator no-op. You can make a copy of this frame to create a new Macro frame)"
        n144 = call <vilib>:"Add State(s) to Queue__jki_lib_state_machine.vi"("State(s) in (\"\")"=w321) -> ("States Out"=w320:string)  [unwired: 14 in]
      }
      frame "Macro: Initialize" {
        # "Initialization Macro\n(This is called once, when the VI starts)"
        n145 = call <vilib>:"Add State(s) to Queue__jki_lib_state_machine.vi"("State(s) in Front (\"\")"="Data: Initialize\nInitialize Core Data\nUI: Initialize\nUI: Update Device List\nUI: Get Device Name\nUI: Start SuperGUI\nUI: Front Panel State >> Open", "State(s) in (\"\")"=w326) -> ("States Out"=w325:string)  [unwired: 13 in]
      }
      frame "Macro: Exit" {
        # "Exit Macro\n(This is called once, when the VI exits)"
        n146 = Unbundle By Name(w333) -> ("Core.Close Panel on Exit?"=w332:bool)
        n147 = Select(t="UI: Front Panel State >> Close", s=w332, f="") -> (s? t:f=w329:string)
        n148 = call <vilib>:"Add State(s) to Queue__jki_lib_state_machine.vi"("State(s) in (\"\")"=w329, "State(s) at Back (\"\")"="Data: Cleanup\nExit") -> ("States Out"=w327:string)  [unwired: 13 in]
        n149 = call <vilib>:"Add State(s) to Queue__jki_lib_state_machine.vi"("State(s) in Front (\"\")"=w327, "State(s) in (\"\")"=w336) -> ("States Out"=w335:string)  [unwired: 13 in]
      }
      frame "---------- New Category ----------" {
        # "Template Separator\n(You can make a copy of, or modify, this frame)"
        n150 = call <vilib>:"Add State(s) to Queue__jki_lib_state_machine.vi"("State(s) in (\"\")"=w340) -> ("States Out"=w339:string)  [unwired: 14 in]
      }
      frame "New Category: 1" {
        # "Your code here.\n(You can make a copy of, or modify, this frame)"
        n151 = call <vilib>:"Add State(s) to Queue__jki_lib_state_machine.vi"("State(s) in (\"\")"=w344) -> ("States Out"=w343:string)  [unwired: 14 in]
      }
      frame "New Category: 2" {
        # "Your code here.\n(You can make a copy of, or modify, this frame)"
        n152 = call <vilib>:"Add State(s) to Queue__jki_lib_state_machine.vi"("State(s) in (\"\")"=w348) -> ("States Out"=w347:string)  [unwired: 14 in]
      }
    }
  }
